vi "Coffee_Random_Price_Generator (SubVI).vi"() -> (2 "String":string, 3 "number":dbl)   [LabVIEW 2019]
uses:
  <vilib>/numeric/Random Number (Range) DBL.vi
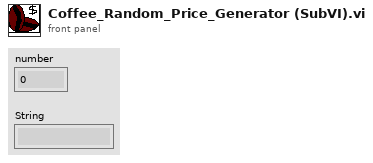
[diagram p1: front panel]
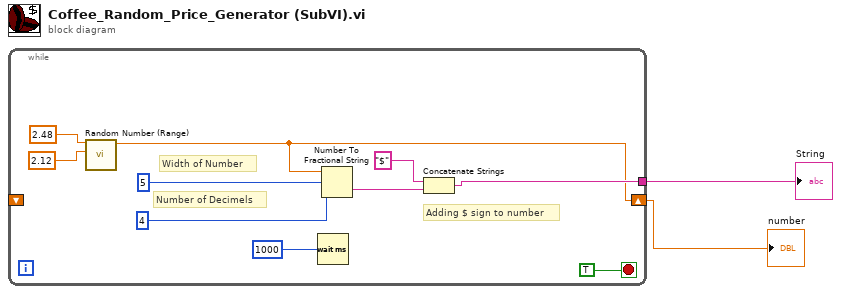
[diagram p0: block diagram]
diagram:
  n1 = while {
    tunnel: [w5] -> w1
    shift-right: [w3] -> w2
    shift-left: _ -> [_]
    stop <- TRUE stop-if-true
    # "Adding $ sign to number"
    # "Number of Decimels"
    # "Width of Number"
    n2 = call-poly <vilib>:"Random Number (Range).vi"("lower bound (0)"=2.12, "upper bound (100)"=2.48) -> ("number"=w3:dbl)  [unwired: 9 in]
    n3 = Wait (ms)(milliseconds to wait=1000) -> ()  [unwired: 1 out]
    n4 = Number To Fractional String(number=w3, width (-)=i16 5, precision (6)=4) -> (F-format string=w9:string)  [unwired: 1 in]
    n5 = Concatenate Strings("$" ("string"), w9) -> (w5:string)
  }
  "number" <- w2
  "String" <- w1
